vi "CleanUp.vi"(8 "error in (no error)":errorcluster, 11 "reference in":refnum<class "WaitOnTestComplete.lvclass">) -> (0 "error out":errorcluster, 3 "reference out":refnum<class "WaitOnTestComplete.lvclass">)   [LabVIEW 2013, in "WaitOnTestComplete.lvclass"]
uses:
  WaitOnTestComplete.lvclass
  Classes/TestCase/TestCase.lvclass
panel:
  # "Copyright © 2007 James Kring, Inc. All rights reserved.\n\nAuthor: Jim Kring [jim.kring@jameskring.com]\n\nThis library is provided \"AS IS\" ,WITHOUT WARRANTIES OR \nCONDITIONS OF ANY KIND, either express or implied.\n\nJames Kring, Inc. -- http://www.jameskring.com"
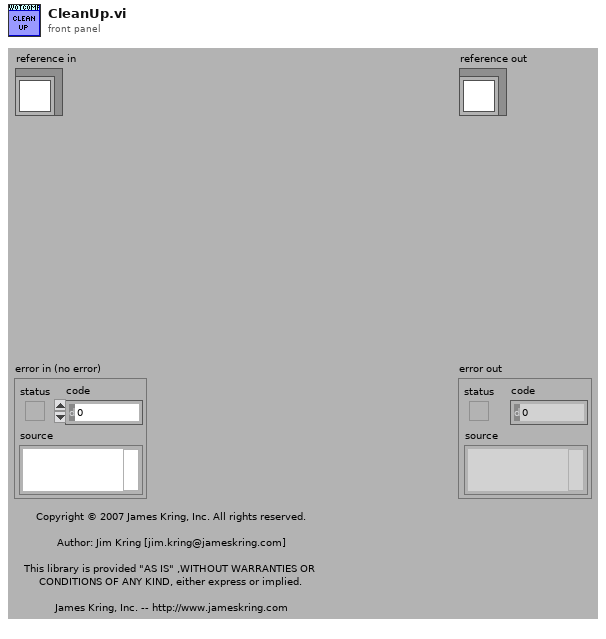
[diagram p1: front panel]
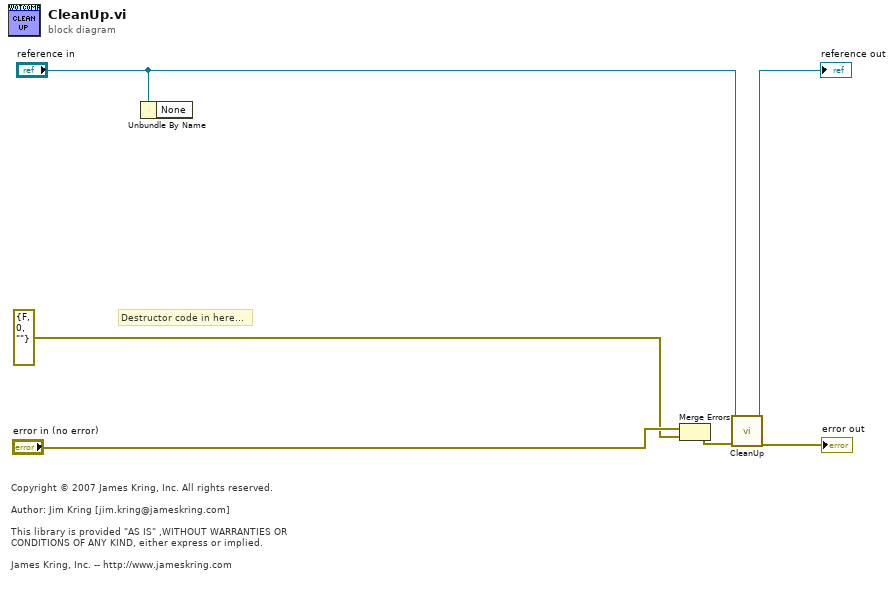
[diagram p0: block diagram]
diagram:
  # "Copyright © 2007 James Kring, Inc. All rights reserved.\n\nAuthor: Jim Kring [jim.kring@jameskring.com]\n\nThis library is provided \"AS IS\" ,WITHOUT WARRANTIES OR \nCONDITIONS OF ANY KIND, either express or implied.\n\nJames Kring, Inc. -- http://www.jameskring.com"
  # "Destructor code in here..."
  n1 = Unbundle By Name("reference in") -> ()  [unwired: 1 out]
  n2 = Merge Errors("error in (no error)", errorcluster {"status"=FALSE, "code"=0, "source"=""} ("error in (no error)")) -> (w2:errorcluster)
  n3 = call-parent "CleanUp.vi"("error in (no error)"=w2, "TestCase in"="reference in") -> ("error out"=→"error out":errorcluster, "TestCase out"=→"reference out":refnum<class "WaitOnTestComplete.lvclass">)  [unwired: 8 in]
